vi "Get Virtual Axis Info.vi"(8 "error in (no error)":errorcluster, 9 "Device Number":string, 10 "Virtual Axis Number (1)":u8=1, 11 "VISA resource name":refnum<visa-resource-name>) -> (0 "error out":errorcluster, 1 "Angle or Ratios":i32[](array[numeric]), 2 "Physical Axes":i32[](array[numeric]), 3 "VISA resource name out":refnum<visa-resource-name>, 4 "Maximum Speed (32-bit)":i32, 5 "Maximum Speed (64-bit)":i64)   [LabVIEW 2018, in "Zaber A Series.lvlib"]
doc: "Returns information about a virtual axis. It returns the numbers of the physical axes incorporated in the virtual axis, the angle or ratio between them, and the maximum speed of the virtual axis in device velocity units.\n\nThe angle/ratio output depends on how the virtual axis was initialized. If the virtual axis was created using an angle, the angle/ratio output will have one entry which is the angle. If ratio setup was used, the output will have multiple entries which are the ratio values.\n\nThis VI requires that the Initialize VI has been called with the same serial port and that the specified virtual axis exists."
uses:
  Zaber A Series.lvlib
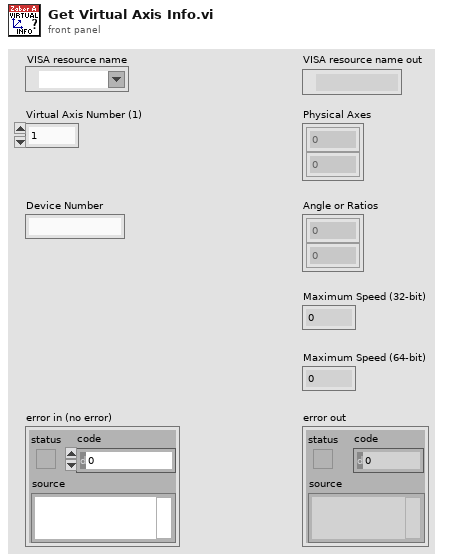
[diagram p1: front panel]
types:
  T1 = cluster{"Device":string, "Axis":string, "Reply Flag":string, "Status":string, "Warning Flags":string, "Data":string}
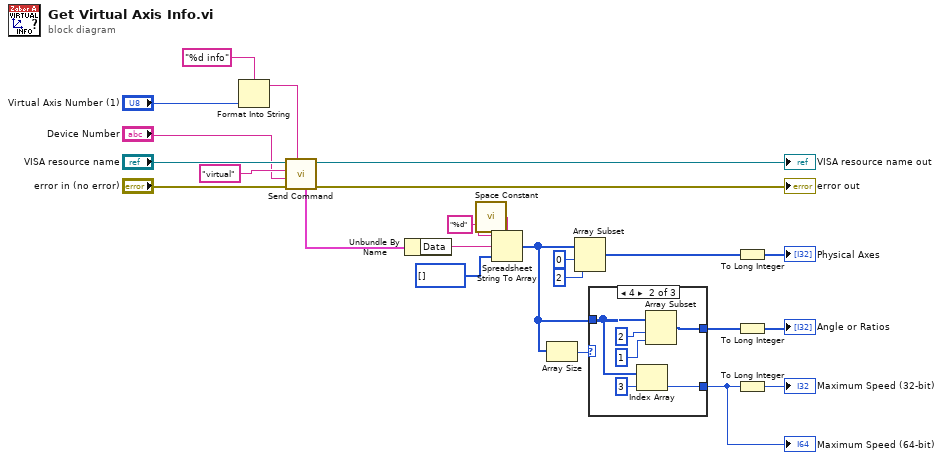
[diagram p0: block diagram]
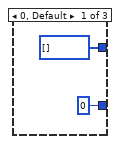
[diagram p2: hidden frame]
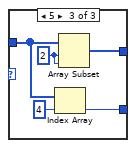
[diagram p3: hidden frame]
diagram:
  n1 = Format Into String(format string="%d info", "Virtual Axis Number (1)") -> (resulting string=w8:string)  [unwired: 2 in, 1 out]
  n2 = call "Send Command.vi"("Data"=w8, "error in (no error)"="error in (no error)", "Device and Axis"="Device Number", "Command"="virtual", "VISA resource name"="VISA resource name") -> ("error out"=→"error out":errorcluster, "VISA resource name out"=→"VISA resource name out":refnum<visa-resource-name>, "First Response Bundle"=w1:T1)  [unwired: 1 in, 3 out]
  n3 = Unbundle By Name(w1) -> ("Data"=w20:string)
  n4 = call <vilib>:"Space Constant.vi"() -> ("String"=w21:string)
  n5 = Spreadsheet String To Array(delimiter (Tab)=w21, format string="%d", spreadsheet string=w20, array type (2D Dbl)=i64[] []) -> (array=w14:i64[])
  n6 = Array Size(array=w14) -> (size(s)=w17:i32)
  n7 = Array Subset(array=w14, index=0, length=2) -> (w7:i64[])
  n8 = case shown="4" w17 {
    tunnel: w14 -> [_ w30 w35]
    tunnel: [i32[] [] w28 w37] -> w5
    tunnel: [0 w31 w33] -> w3
    frame 0, Default {
    }
    frame 4 {
      n9 = Index Array(array=w30, index=3) -> (element=w31:i64)
      n10 = Array Subset(array=w30, index=2, length=1) -> (w28:i64[])
    }
    frame 5 {
      w36 = 2 ("index")
      n11 = Index Array(array=w35, index=4) -> (element=w33:i64)
      n12 = Array Subset(array=w35, index=w36, length=w36) -> (w37:i64[])
    }
  }
  "Maximum Speed (64-bit)" <- w3
  n13 = To Long Integer(number=w7) -> (32bit integer=→"Physical Axes":i32[])
  n14 = To Long Integer(number=w5) -> (32bit integer=→"Angle or Ratios":i32[])
  n15 = To Long Integer(number=w3) -> (32bit integer=→"Maximum Speed (32-bit)":i32)
